vi "FRC-Traj-Lib-analog-adv-pid-complex-test.vi"() -> ()   [LabVIEW 2019]
uses:
  <vilib>/Rock Robotics/WPI/ThirdParty/JAS_Junk/TrajLib/PID_CONTROLLER.ctl
  <vilib>/Rock Robotics/WPI/ThirdParty/JAS_Junk/TrajLib/LinearFilter_ResetToValue.vi
  <vilib>/Rock Robotics/WPI/ThirdParty/JAS_Junk/TrajLib/LinearFilter_Calculate.vi
  <vilib>/Rock Robotics/WPI/ThirdParty/JAS_Junk/TrajLib/PIDController_AtSetpoint.vi
  <vilib>/Rock Robotics/WPI/ThirdParty/JAS_Junk/TrajLib/PIDController_SetPIDF.vi
  <vilib>/Rock Robotics/WPI/ThirdParty/JAS_Junk/TrajLib/PIDController_SetDerivativeFilter.vi
  <vilib>/Rock Robotics/WPI/ThirdParty/JAS_Junk/TrajLib/PIDController_SetIntegratorRange.vi
  <vilib>/Rock Robotics/WPI/ThirdParty/JAS_Junk/TrajLib/PIDController_SetTolerancePandV.vi
  <vilib>/Rock Robotics/WPI/ThirdParty/JAS_Junk/TrajLib/PIDController_DisableContinousInput.vi
  <vilib>/Rock Robotics/WPI/ThirdParty/JAS_Junk/TrajLib/PIDController_SetInputRange.vi
  <vilib>/Rock Robotics/WPI/ThirdParty/JAS_Junk/TrajLib/PIDController_EnableContinousInput.vi
  <vilib>/Rock Robotics/WPI/ThirdParty/JAS_Junk/TrajLib/PIDController_Reset.vi
  <vilib>/Rock Robotics/WPI/ThirdParty/JAS_Junk/TrajLib/PIDController_New.vi
  <vilib>/Rock Robotics/WPI/ThirdParty/JAS_Junk/TrajLib/PIDController_SetOutputLimits.vi
  <vilib>/Rock Robotics/WPI/ThirdParty/JAS_Junk/TrajLib/PIDController_NewPeriod.vi
  <vilib>/Rock Robotics/SystemInterfaces/NetworkCommunication/NetComm_UsageReport_report.vi
  <vilib>/Rock Robotics/WPI/ThirdParty/JAS_Junk/TrajLib/Util_LibraryGlobals.vi
  <vilib>/Rock Robotics/WPI/ThirdParty/JAS_Junk/TrajLib/PIDController_AdvCalculate_FF_Sp_Pv.vi
  <vilib>/addons/control/pid/pid.llb/PID Lead-Lag (DBL).vi
  <vilib>/Rock Robotics/WPI/ThirdParty/JAS_Junk/TrajLib/LinearFilter_MovingAverage.vi
  <vilib>/Rock Robotics/WPI/ThirdParty/JAS_Junk/TrajLib/LinearFilter_LowPassBW1.vi
  <vilib>/Rock Robotics/WPI/ThirdParty/JAS_Junk/TrajLib/LinearFilter_LowPassBW2.vi
  <vilib>/Rock Robotics/WPI/ThirdParty/JAS_Junk/TrajLib/LinearFilter_HighPassBW1.vi
  <vilib>/Rock Robotics/WPI/ThirdParty/JAS_Junk/TrajLib/LinearFilter_HighPassBW2.vi
  <vilib>/addons/control/pid/NI_PID_pid.lvlib
  <vilib>/Rock Robotics/WPI/ThirdParty/JAS_Junk/TrajLib/Trajectory_Library.lvlib
panel:
  in  "Desired Speed":dbl(slide)=-0.22222222222222499 scale=-50.0..50.0 scale format="%#.1f"
  in  "Tab Control":T1(tab)
  in  "Enable Noise":bool=TRUE
  in  "Auto / Manual":bool=TRUE
  out "Dash Speed Demand":dbl format="%10.2f"
  out "Dash Speed Target":dbl format="%10.2f"
  out "DashRightMotorOutput":dbl format="%11.3f"
  out "DashRight Wheel Speed":dbl(knob)=-2.895988890827539e-05 scale=-60.0..60.0
  out "Right Wheel ErrorFilt":dbl format="%11.3f"
  out "Right Wheel SpeedFilt":dbl format="%10.2f"
  out "DashLeft Wheel Speed":dbl(knob)=-2.895988890827539e-05 scale=-60.0..60.0
  out "Left Wheel ErrorFilt":dbl format="%11.3f"
  out "DashLeftMotorOutput":dbl format="%11.3f"
  out "Left Wheel Speed Filt":dbl format="%10.2f"
  out "Duration":dbl format="%11.3f"
  out "Late":dbl format="%11.3f"
  out "SP, PV, CO Left":T2(graph)
  out "SP, PV, CO Right":T2(graph)
  in  "SetPoint Change Rate":dbl=80.0 min=1.0 max=9000.0 format="%14.4f"
  in  "Right PID Error Tolerance":T3={"PositionTolerance"=0.001, "VelocityTolerance"=9.9e+30}
  in  "Right Adv PID Limits":T4={"MaxInput"=50.0, "MinInput"=-50.0, "Continuous"=FALSE, "MaxOutput"=1.0, "MinOutput"=-1.0}
  in  "Left Adv PID Limits":T4={"MaxInput"=50.0, "MinInput"=-50.0, "Continuous"=FALSE, "MaxOutput"=1.0, "MinOutput"=-1.0}
  in  "Left PID Error Tolerance":T3={"PositionTolerance"=0.001, "VelocityTolerance"=9.9e+30}
  in  "Left Adv PID Tuning":T5={"Kf"=0.02, "Kp"=0.06, "Ki"=0.1, "Kd"=0.004, "MaximumIntegral"=9.9e+30, "MinimumIntegral"=-9.9e+30, "Filter Derivative"=TRUE}
  in  "Right Adv PID Tuning":T5={"Kf"=0.02, "Kp"=0.06, "Ki"=0.1, "Kd"=0.004, "MaximumIntegral"=9.9e+30, "MinimumIntegral"=-9.9e+30, "Filter Derivative"=TRUE}
  out "Left PID Data":T6={"Kp"=0.0, "Ki"=0.0, "Kd"=0.0, "Period"=0.0, "Max_Integral"=0.0, "Min_Integral"=0.0, "Max_Input"=0.0, "Min_Input"=0.0, "Input_Range"=0.0, "Continuous"=FALSE, "PositionError"=0.0, "VelocityError"=0.0, "PrevError"=0.0, "TotalError"=0.0, "PositionTolerance"=0.0, "VelocityTolerance"=0.0, "SetPoint"=0.0, "Kf"=0.0, "Prev_Deriv"=0.0, "Prev_Deriv 2"=0.0, "DerivativeFilter"=FALSE, "Min_Output"=-9.99e+35, "Max_Output"=9.9e+35, "Prev_F_P"=0.0, "Prev_F_P_2"=0.0, "AntiWindupActive"=FALSE} {"Prev_F_P_2" format="%16_6e"; "Prev_F_P" format="%16_6e"; "Max_Output" format="%16_6e"; "Min_Output" format="%16_6e"; "Prev_Deriv 2" format="%16_6e"; "Prev_Deriv" format="%16_6e"; "Kf" format="%16_6e"; "SetPoint" format="%17.6f"; "VelocityTolerance" format="%17.6f"; "PositionTolerance" format="%17.6f"; "TotalError" format="%17.6f"; "PrevError" format="%17.6f"; "VelocityError" format="%17.6f"; "PositionError" format="%17.6f"; "Input_Range" format="%17.6f"; "Min_Input" format="%17.6f"; "Max_Input" format="%17.6f"; "Min_Integral" format="%17.6f"; "Max_Integral" format="%17.6f"; "Period" format="%17.6f"; "Kd" format="%17.6f"; "Ki" format="%17.6f"; "Kp" format="%17.6f"}
  out "Right PID Data":T6={"Kp"=0.0, "Ki"=0.0, "Kd"=0.0, "Period"=0.0, "Max_Integral"=0.0, "Min_Integral"=0.0, "Max_Input"=0.0, "Min_Input"=0.0, "Input_Range"=0.0, "Continuous"=FALSE, "PositionError"=0.0, "VelocityError"=0.0, "PrevError"=0.0, "TotalError"=0.0, "PositionTolerance"=0.0, "VelocityTolerance"=0.0, "SetPoint"=0.0, "Kf"=0.0, "Prev_Deriv"=0.0, "Prev_Deriv 2"=0.0, "DerivativeFilter"=FALSE, "Min_Output"=-9.99e+35, "Max_Output"=9.9e+35, "Prev_F_P"=0.0, "Prev_F_P_2"=0.0, "AntiWindupActive"=FALSE} {"Prev_F_P_2" format="%16_6e"; "Prev_F_P" format="%16_6e"; "Max_Output" format="%16_6e"; "Min_Output" format="%16_6e"; "Prev_Deriv 2" format="%16_6e"; "Prev_Deriv" format="%16_6e"; "Kf" format="%16_6e"; "SetPoint" format="%17.6f"; "VelocityTolerance" format="%17.6f"; "PositionTolerance" format="%17.6f"; "TotalError" format="%17.6f"; "PrevError" format="%17.6f"; "VelocityError" format="%17.6f"; "PositionError" format="%17.6f"; "Input_Range" format="%17.6f"; "Min_Input" format="%17.6f"; "Max_Input" format="%17.6f"; "Min_Integral" format="%17.6f"; "Max_Integral" format="%17.6f"; "Period" format="%17.6f"; "Kd" format="%17.6f"; "Ki" format="%17.6f"; "Kp" format="%17.6f"}
  in  "RightWheelNoise":dbl
  in  "LeftWheelNoise":dbl
  out "RightWheelSpeed":dbl
  out "LeftWheelSpeed":dbl
  out "RightMotorOutput":dbl
  out "LeftMotorOutput":dbl
  out "SpeedSetpoint":dbl
  in  "SpeedTarget":dbl
  in  "SpeedControlEnabled":bool
  out "LibUsage_Kinematics":i32 format="%20.0f"
  out "LibUsage_TrapezoidProfile":i32 format="%20.0f"
  out "LibUsage_LinearFIlter":i32 format="%20.0f"
  out "LibUsage_Odometry":i32 format="%20.0f"
  out "LibUsage_PIDController":i32 format="%20.0f"
  out "LibUsage_ProfiledPID":i32 format="%20.0f"
  # "Enter a desired speed and then press the Set Speed Target \nbutton.  This simulates the joystick input."
  # "FT/SEC"
  # "Example of Closed Loop Motor Speed Control\nUses Advanced PID"
  # "This value shows the current speed of each wheel.  This is measured by an encoder.  The encoder measures\n speed by counting pulses of the wheel turning and dividing by the time interval.  Total distance change\nis also a result.  This value is called the \"Process Variable\"."
  # "FT/SEC"
  # "FT/SEC"
  # "FT/SEC"
  # "The Speed Target is rate limited so not to make\nto drastic a change in the desired speed.  (This is\nwhat happens mechanically when pushing the gas\npedal of a real car.)"
  # "This error value shows the error between the current speed\nand the speed demand."
  # "FT/SEC"
  # "This example adds a \"Manual\" mode so that the still operates\nif the encoder fails."
  # "FT/SEC"
  # "FT/SEC"
  # "This value shows the current motor output demand.  This could also be a motor speed demand and \nanother closed loop controller would control the motor speed.  In this simple example this value is \nused to drive the simulated motor directly.  This motor demand is called the \"Control Output\"."
  # "Enables some simulated process noise"
  # "FT/SEC/SEC"
  # "These are the tuning parameters for the PID VI"
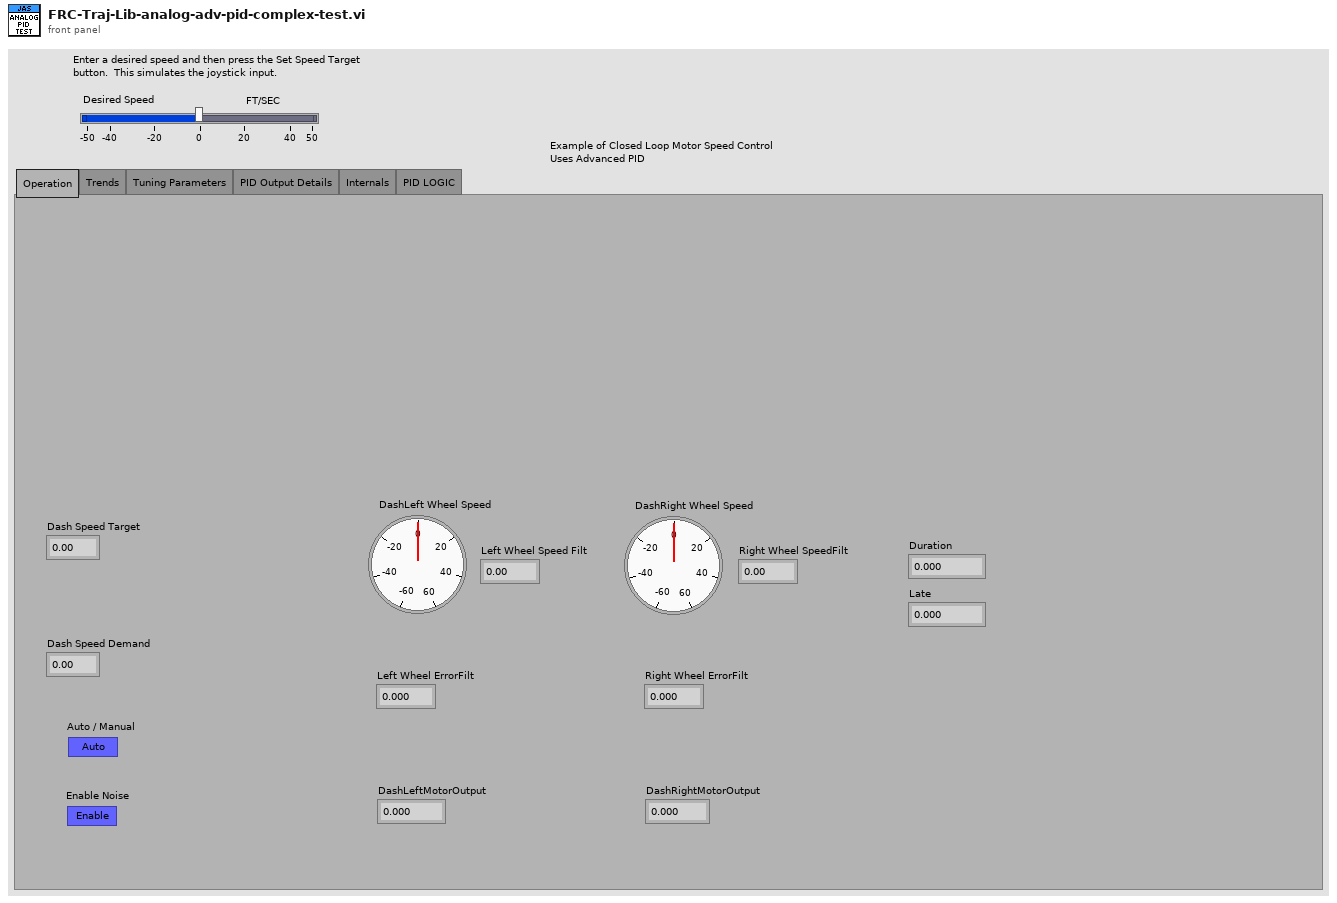
[diagram p1: front panel]
types:
  T1 = enum32{"Operation", "Trends", "Tuning Parameters", "PID Output Details", "Internals", "PID LOGIC"}
  T2 = cluster{"MotorDemand":dbl, "CurrentSetpoint":dbl, "CurrentPosition":dbl}
  T3 = cluster{"PositionTolerance":dbl, "VelocityTolerance":dbl}
  T4 = cluster{"MaxInput":dbl, "MinInput":dbl, "Continuous":bool, "MaxOutput":dbl, "MinOutput":dbl}
  T5 = cluster{"Kf":dbl, "Kp":dbl, "Ki":dbl, "Kd":dbl, "MaximumIntegral":dbl, "MinimumIntegral":dbl, "Filter Derivative":bool}
  T6 = typedef "Trajectory_Library.lvlib/PID_CONTROLLER.ctl" = cluster{"Kp":dbl, "Ki":dbl, "Kd":dbl, "Period":dbl, "Max_Integral":dbl, "Min_Integral":dbl, "Max_Input":dbl, "Min_Input":dbl, "Input_Range":dbl, "Continuous":bool, "PositionError":dbl, "VelocityError":dbl, "PrevError":dbl, "TotalError":dbl, "PositionTolerance":dbl, "VelocityTolerance":dbl, "SetPoint":dbl, "Kf":dbl, "Prev_Deriv":dbl, "Prev_Deriv 2":dbl, "DerivativeFilter":bool, "Min_Output":dbl, "Max_Output":dbl, "Prev_F_P":dbl, "Prev_F_P_2":dbl, "AntiWindupActive":bool}
  T7 = cluster{"gain":dbl, "lag time":dbl, "lead time":dbl}
  T8 = enum16{"Moving Average", "Low Pass 1st Order Butterworth", "Low Pass 2nd Order Butterworth", "High Pass 1st Order Butterworth", "High Pass 2nd Order Butterworth"}
  T9 = cluster{"LeftMotorOutput":dbl, "SpeedSetpoint":dbl, "LeftWheelSpeed":dbl}
  T10 = cluster{"RightMotorOutput":dbl, "SpeedSetpoint":dbl, "RightWheelSpeed":dbl}
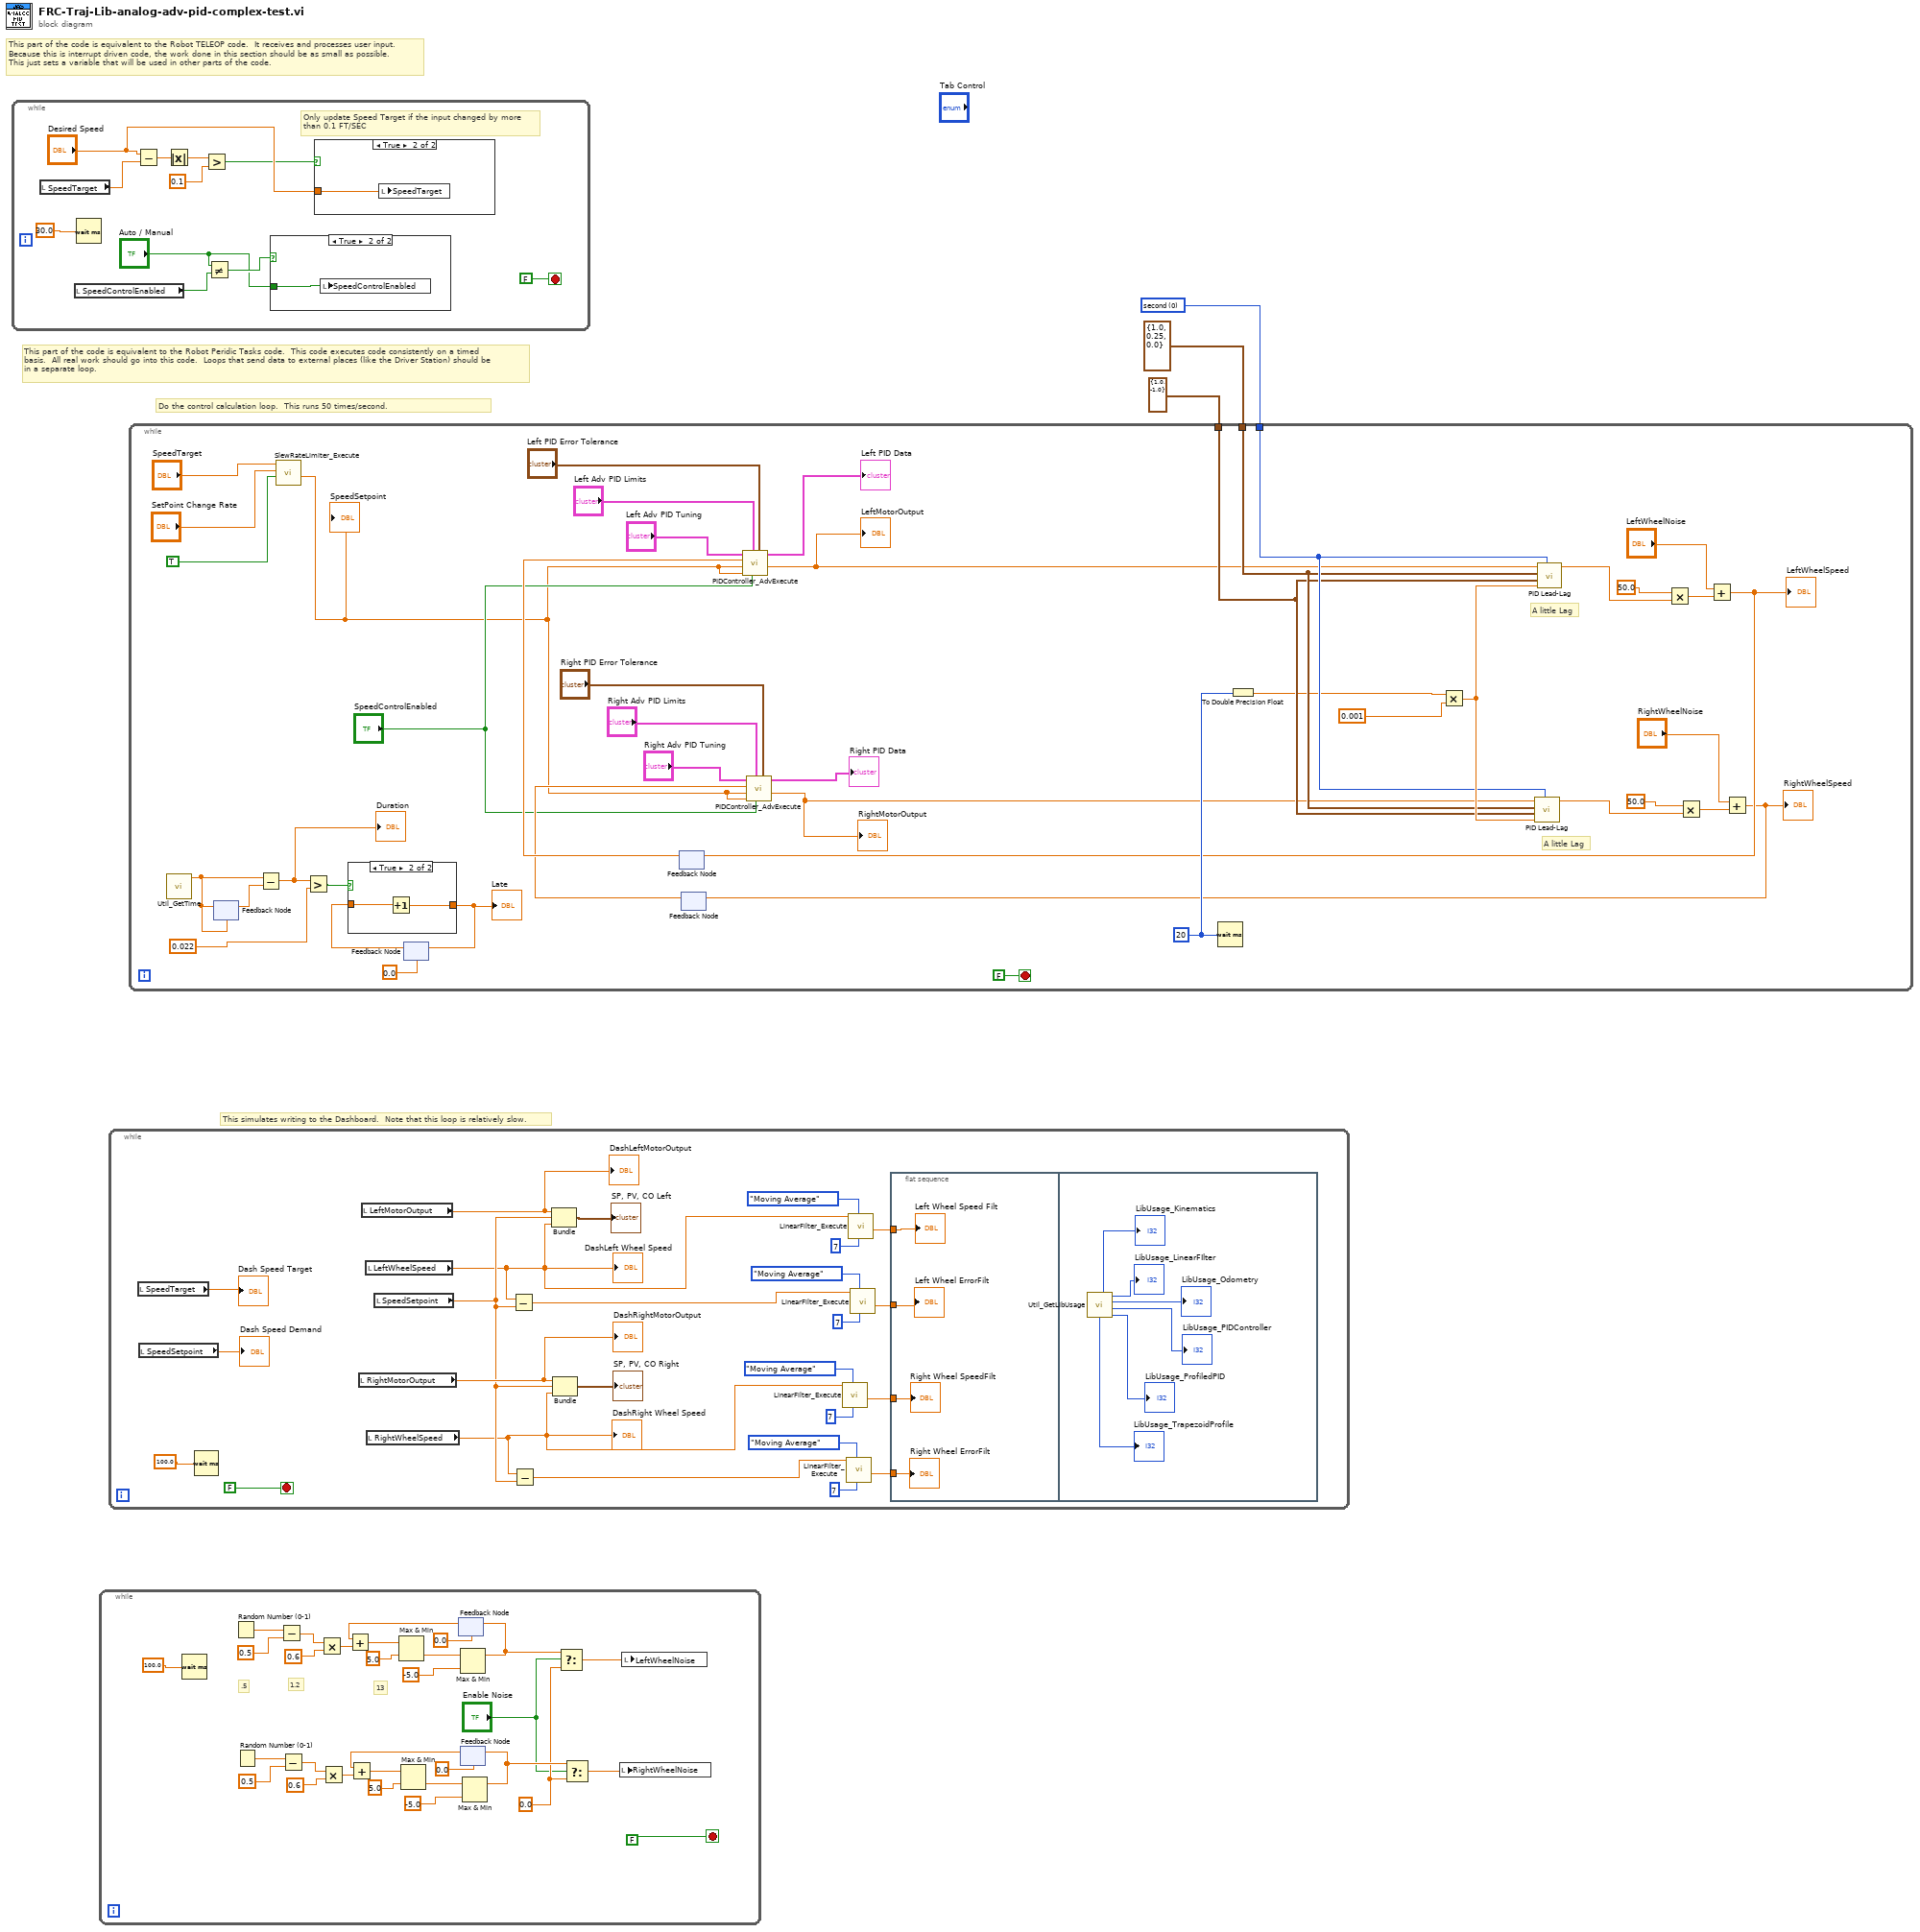
[diagram p0: block diagram]
diagram:
  w3 = u16 0 items=["second", "minute"] ("time unit")
  # "This simulates writing to the Dashboard.  Note that this loop is relatively slow."
  # "Do the control calculation loop.  This runs 50 times/second."
  # "This part of the code is equivalent to the Robot Peridic Tasks code.  This code executes code consistently on a timed\nbasis.  All real work should go into this code.  Loops that send data to external places (like the Driver Station) should be \nin a separate loop."
  # "This part of the code is equivalent to the Robot TELEOP code.  It receives and processes user input.\nBecause this is interrupt driven code, the work done in this section should be as small as possible.\nThis just sets a variable that will be used in other parts of the code."
  n1 = while {
    stop <- FALSE stop-if-true
    # "Only update Speed Target if the input changed by more\nthan 0.1 FT/SEC"
    n2 = local read "SpeedTarget"() -> (w13:dbl)
    n3 = local read "SpeedControlEnabled"() -> (w5:bool)
    n4 = Wait (ms)(milliseconds to wait=30.0) -> ()  [unwired: 1 out]
    n5 = Subtract(x="Desired Speed", y=w13) -> (x-y=w12:dbl)
    n6 = Absolute Value(x=w12) -> (abs(x)=w11:dbl)
    n7 = Greater?(x=w11, y=0.1) -> (0:w8:bool)
    n8 = Not Equal?(x="Auto / Manual", y=w5) -> (x != y?=w6:bool)
    n9 = case shown="True" w6 {
      tunnel: "Auto / Manual" -> [_ w15]
      frame False {
      }
      frame True {
        n10 = local write "SpeedControlEnabled"(w15) -> ()
      }
    }
    n11 = case shown="True" w8 {
      tunnel: "Desired Speed" -> [_ w16]
      frame False {
      }
      frame True {
        n12 = local write "SpeedTarget"(w16) -> ()
      }
    }
  }
  n13 = while {
    stop <- FALSE stop-if-true
    w20 = 0.0 ("f")
    # "13"
    # "1.2"
    # ".5"
    n14 = Wait (ms)(milliseconds to wait=100.0) -> ()  [unwired: 1 out]
    n15 = Random Number (0-1)() -> (number: 0 to 1=w18:dbl)
    n16 = Random Number (0-1)() -> (number: 0 to 1=w17:dbl)
    n17 = Subtract(x=w18, y=0.5) -> (x-y=w37:dbl)
    n18 = Subtract(x=w17, y=0.5) -> (x-y=w27:dbl)
    n19 = Multiply(x=w37, y=0.6) -> (x*y=w36:dbl)
    n20 = Multiply(x=w27, y=0.6) -> (x*y=w26:dbl)
    n21 = feedback #1(0.0) -> (w39:dbl)
    n22 = Add(x=w39, y=w36) -> (x+y=w43:dbl)
    n23 = Max & Min(x=w43, y=5.0) -> (min(x,y)=w42:dbl)  [unwired: 1 out]
    n24 = Max & Min(x=w42, y=-5.0) -> (max(x,y)=w23:dbl)  [unwired: 1 out]
    n25 = feedback-in #1(w23) -> ()
    n26 = feedback #2(0.0) -> (w29:dbl)
    n27 = Add(x=w29, y=w26) -> (x+y=w33:dbl)
    n28 = Max & Min(x=w33, y=5.0) -> (min(x,y)=w32:dbl)  [unwired: 1 out]
    n29 = Max & Min(x=w32, y=-5.0) -> (max(x,y)=w21:dbl)  [unwired: 1 out]
    n30 = feedback-in #2(w21) -> ()
    n31 = Select(t=w23, s="Enable Noise", f=w20) -> (s? t:f=w24:dbl)
    n32 = Select(t=w21, s="Enable Noise", f=w20) -> (s? t:f=w22:dbl)
    n33 = local write "RightWheelNoise"(w22) -> ()
    n34 = local write "LeftWheelNoise"(w24) -> ()
  }
  n35 = while {
    stop <- FALSE stop-if-true
    n36 = local read "SpeedTarget"() -> (→"Dash Speed Target":dbl)
    n37 = local read "SpeedSetpoint"() -> (→"Dash Speed Demand":dbl)
    n38 = Wait (ms)(milliseconds to wait=100.0) -> ()  [unwired: 1 out]
    n39 = local read "RightMotorOutput"() -> (w67:dbl)
    "DashRightMotorOutput" <- w67
    n40 = local read "LeftMotorOutput"() -> (w64:dbl)
    "DashLeftMotorOutput" <- w64
    n41 = local read "LeftWheelSpeed"() -> (w60:dbl)
    "DashLeft Wheel Speed" <- w60
    n42 = local read "RightWheelSpeed"() -> (w51:dbl)
    "DashRight Wheel Speed" <- w51
    n43 = local read "SpeedSetpoint"() -> (w63:dbl)
    n44 = Subtract(x=w60, y=w63) -> (x-y=w56:dbl)
    n45 = Subtract(x=w51, y=w63) -> (x-y=w47:dbl)
    n46 = Bundle("LeftMotorOutput"=w64, "SpeedSetpoint"=w63, "LeftWheelSpeed"=w60) -> (→"SP, PV, CO Left":T9)  [unwired: 1 in]
    n47 = Bundle("RightMotorOutput"=w67, "SpeedSetpoint"=w63, "RightWheelSpeed"=w51) -> (→"SP, PV, CO Right":T10)  [unwired: 1 in]
    n48 = call <vilib>:"LinearFilter_Execute.vi"("Samples"=7, "Filter Type"=T8."Moving Average", "Input"=w51) -> ("Output"=w52:dbl)  [unwired: 7 in, 1 out]
    n49 = call <vilib>:"LinearFilter_Execute.vi"("Samples"=7, "Filter Type"=T8."Moving Average", "Input"=w47) -> ("Output"=w48:dbl)  [unwired: 7 in, 1 out]
    n50 = call <vilib>:"LinearFilter_Execute.vi"("Samples"=7, "Filter Type"=T8."Moving Average", "Input"=w60) -> ("Output"=w59:dbl)  [unwired: 7 in, 1 out]
    n51 = call <vilib>:"LinearFilter_Execute.vi"("Samples"=7, "Filter Type"=T8."Moving Average", "Input"=w56) -> ("Output"=w55:dbl)  [unwired: 7 in, 1 out]
    n52 = flat-sequence {
      tunnel: w59 -> [w75]
      tunnel: w55 -> [w74]
      tunnel: w52 -> [w73]
      tunnel: w48 -> [w72]
      frame #0 {
        "Left Wheel ErrorFilt" <- w74
        "Right Wheel ErrorFilt" <- w72
        "Left Wheel Speed Filt" <- w75
        "Right Wheel SpeedFilt" <- w73
      }
      frame #1 {
        n53 = call <vilib>:"Util_GetLibUsage.vi"() -> ("LibUsage_ProfiledPID"=→"LibUsage_ProfiledPID":i32, "LibUsage_PIDController"=→"LibUsage_PIDController":i32, "LibUsage_Odometry"=→"LibUsage_Odometry":i32, "LibUsage_LinearFIlter"=→"LibUsage_LinearFIlter":i32, "LibUsage_TrapezoidProfile"=→"LibUsage_TrapezoidProfile":i32, "LibUsage_Kinematics"=→"LibUsage_Kinematics":i32)  [unwired: 6 in]
      }
    }
  }
  n54 = while {
    tunnel: w3 -> [w101]
    tunnel: T7 {"gain"=1.0, "lag time"=0.25, "lead time"=0.0} ("tuning parameters") -> [w100]
    tunnel: cluster{"output high":dbl, "output low":dbl} {"output high"=1.0, "output low"=-1.0} ("output range") -> [w99]
    stop <- FALSE stop-if-true
    w98 = u32 20 ("milliseconds to wait")
    # "A little Lag"
    # "A little Lag"
    n55 = call <vilib>:"Util_GetTime.vi"() -> ("FPGA_Time_Seconds"=w117:dbl)  [unwired: 9 in, 2 out]
    n56 = feedback #3(w117) -> (w116:dbl)
    n57 = feedback-in #3(w117) -> ()
    n58 = Subtract(x=w117, y=w116) -> (x-y=w114:dbl)
    "Duration" <- w114
    n59 = call <vilib>:"SlewRateLimiter_Execute.vi"("Enable"=TRUE, "Rate"="SetPoint Change Rate", "Input"="SpeedTarget") -> ("Output"=w85:dbl)  [unwired: 7 in, 1 out]
    "SpeedSetpoint" <- w85
    n60 = Greater?(x=w114, y=0.022) -> (0:w115:bool)
    n61 = feedback #4(0.0) -> (w118:dbl)
    n62 = case shown="True" w115 {
      tunnel: [w125 w127] -> w119
      tunnel: w118 -> [w125 w126]
      frame False {
      }
      frame True {
        n63 = Increment(x=w126) -> (x+1=w127:dbl)
      }
    }
    "Late" <- w119
    n64 = feedback-in #4(w119) -> ()
    n65 = feedback #5() -> (w94:dbl)  [unwired: 1 in]
    n66 = feedback #6() -> (w93:dbl)  [unwired: 1 in]
    n67 = call <vilib>:"PIDController_AdvExecute.vi"("PID Error Tolerance"="Left PID Error Tolerance", "Auto"="SpeedControlEnabled", "Adv PID Limits"="Left Adv PID Limits", "FF-FeedForward"=w85, "SP-SetPoint"=w85, "PV-Measurement"=w94, "Adv PID Tuning"="Left Adv PID Tuning") -> ("CO-ControlOutput"=w87:dbl, "out PID_CONTROLLER"=→"Left PID Data":T6)  [unwired: 2 in, 1 out]
    "LeftMotorOutput" <- w87
    n68 = call <vilib>:"PIDController_AdvExecute.vi"("PID Error Tolerance"="Right PID Error Tolerance", "Auto"="SpeedControlEnabled", "Adv PID Limits"="Right Adv PID Limits", "FF-FeedForward"=w85, "SP-SetPoint"=w85, "PV-Measurement"=w93, "Adv PID Tuning"="Right Adv PID Tuning") -> ("CO-ControlOutput"=w88:dbl, "out PID_CONTROLLER"=→"Right PID Data":T6)  [unwired: 2 in, 1 out]
    "RightMotorOutput" <- w88
    n69 = Wait (ms)(milliseconds to wait=w98) -> ()  [unwired: 1 out]
    n70 = To Double Precision Float(number=w98) -> (double precision float=w97:dbl)
    n71 = Multiply(x=w97, y=0.001) -> (x*y=w109:dbl)
    n72 = call-poly <vilib>:"PID Lead-Lag.vi"("time unit"=w101, "dt (s)"=w109, "output range"=w99, "tuning parameters"=w100, "input"=w88) -> ("output"=w92:dbl)  [unwired: 3 in, 1 out]
    n73 = call-poly <vilib>:"PID Lead-Lag.vi"("time unit"=w101, "dt (s)"=w109, "output range"=w99, "tuning parameters"=w100, "input"=w87) -> ("output"=w110:dbl)  [unwired: 3 in, 1 out]
    n74 = Multiply(x=50.0, y=w110) -> (x*y=w106:dbl)
    n75 = Multiply(x=50.0, y=w92) -> (x*y=w105:dbl)
    n76 = Add(x="LeftWheelNoise", y=w106) -> (x+y=w96:dbl)
    "LeftWheelSpeed" <- w96
    n77 = feedback-in #5(w96) -> ()
    n78 = Add(x="RightWheelNoise", y=w105) -> (x+y=w95:dbl)
    "RightWheelSpeed" <- w95
    n79 = feedback-in #6(w95) -> ()
  }
